vi "Cage-get-connect.vi"(8 "error in (no error)":errorcluster, 9 "Cluster in":T1, 11 "reference in":refnum<k24>) -> (0 "error out":errorcluster, 1 "Cluster out":T1, 2 "IsConnected":bool, 3 "reference out":refnum<k24>)   [LabVIEW 2018]
uses:
  Thorlabs Translation Stages/Controls/Translation Stage Cluster.ctl
  General/Controls/Translation Stage Types.ctl
  C:/Project/SSOCT/Labview Software/Thorlabs.MotionControl.Controls.dll
  Thorlabs.MotionControl.Controls.dll
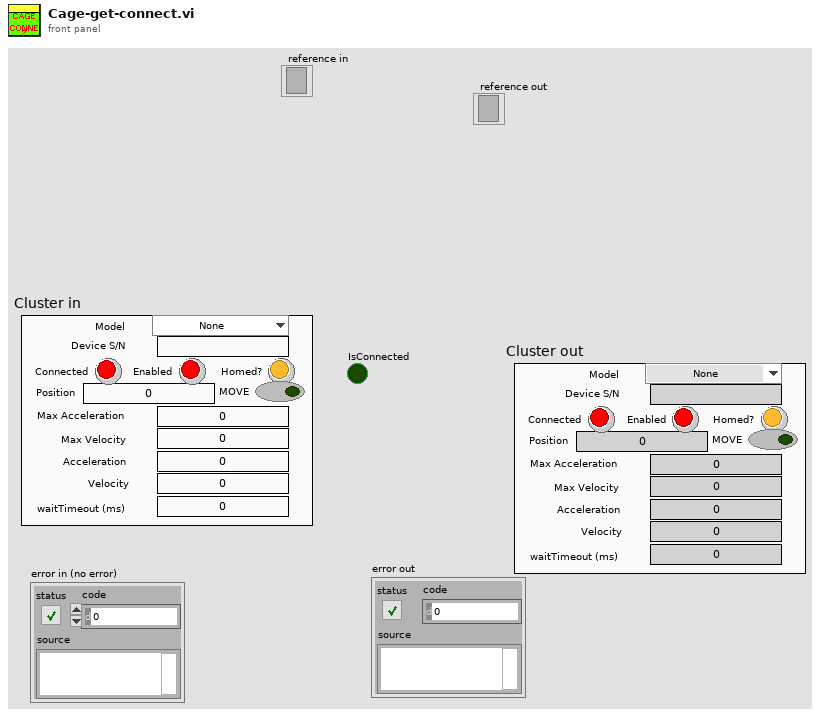
[diagram p1: front panel]
types:
  T1 = typedef "Translation Stage Cluster.ctl" = cluster{"Position":dbl, "Is.Enabled?":bool, "Is.Connected?":bool, "Device SN":string, "AccelerationMaximum":dbl, "VelocityMaximum":dbl, "Acceleration":dbl, "Velocity":dbl, "waitTimeout (ms)":i32, "Model":T2, "Is.Homed?":bool, "MOVE":bool}
  T2 = typedef "Translation Stage Types.ctl" = enum16{"None", "Thorlabs LTS", "Thorlabs MLJ"}
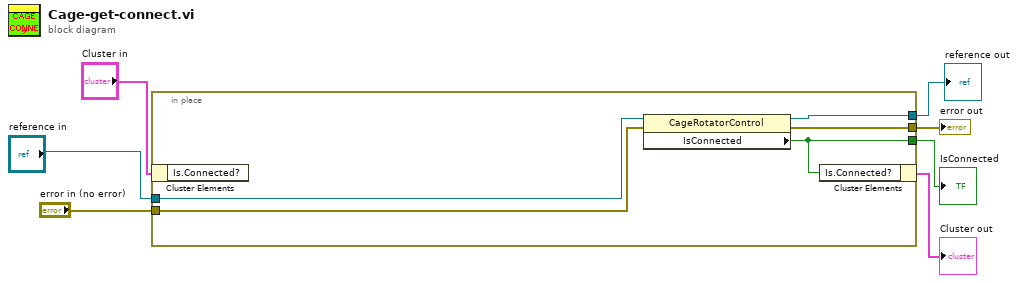
[diagram p0: block diagram]
diagram:
  n1 = in-place {
    in-place-border: "reference in" -> [w8]
    in-place-border: [w12] -> w6
    in-place-border: "error in (no error)" -> [w9]
    in-place-border: [w11] -> w4
    in-place-border: [w10] -> w2
    n2 = in-place-cluster #1("Cluster in") -> ()  [unwired: 1 out]
    n3 = property class="CageRotatorControl"(reference=w8, error in=w9) -> (reference out=w12:refnum<k24>, error out=w11:errorcluster, "IsConnected"=w10:bool)
    n4 = in-place-cluster #1("Is.Connected?"=w10) -> (→"Cluster out":T1)
  }
  "error out" <- w4
  "IsConnected" <- w2
  "reference out" <- w6
